vi "Write ActionVIType.vi"(8 "error in (no error)":errorcluster, 10 "Enum":T1, 11 "ActionVI in":refnum<class "ActionVI.lvclass">) -> (0 "error out":errorcluster, 3 "ActionVI out":refnum<class "ActionVI.lvclass">)   [LabVIEW 2019, in "ActionVI.lvclass"]
uses:
  ActionVI.lvclass
  Controls/ActionVITypes.ctl
  ActionVI.lvclass/ActionVI.ctl
  Configuration Tool.lvlib
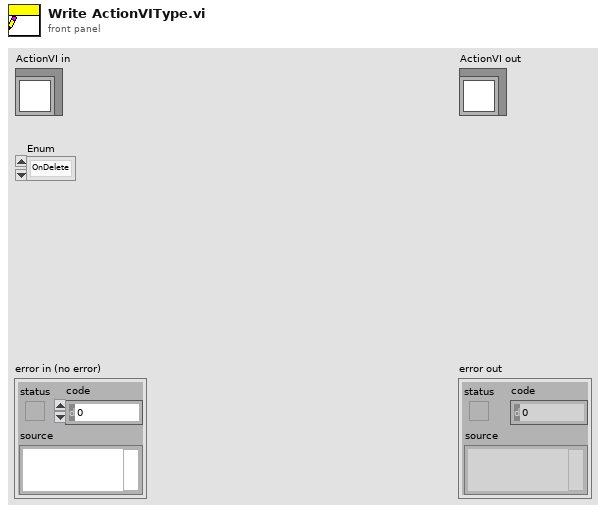
[diagram p1: front panel]
types:
  T1 = typedef "Configuration Tool.lvlib/ActionVITypes.ctl" = enum16{"OnDelete", "OnLoad", "OnPaste", "OnTargetTypeChange", "OnDeleteRequest", "OnCompile", "OnSystemShutdown", "OnSave", "OnDownload"}
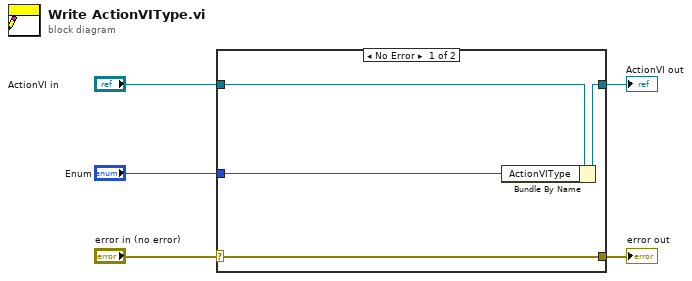
[diagram p0: block diagram]
diagram:
  n1 = case shown="No Error" "error in (no error)" {
    selector: "error in (no error)" -> [w9 w10]
    tunnel: [w9 w10] -> w4
    tunnel: [w7 w11] -> w2
    tunnel: "ActionVI in" -> [w8 w11]
    tunnel: "Enum" -> [w6 _]
    frame No Error {
      n2 = Bundle By Name(cluster=w8, "ActionVIType"=w6) -> (w7:refnum<class "ActionVI.lvclass">)
    }
    frame Error {
    }
  }
  "error out" <- w4
  "ActionVI out" <- w2
